vi "Control Panel.vi"() -> ()   [LabVIEW 2020]
panel:
  in  "Enable/Disable":bool
  out "Panel 8":bool
  out "Panel 7":bool
  out "Panel 6":bool
  out "Panel 5":bool
  out "Panel 4":bool
  out "Panel 3":bool
  out "Panel 2":bool
  out "Panel 1":bool
  out "Holoprojector 3":bool
  out "Holoprojector 2":bool
  out "Holoprojector 1":bool
  out "2D Picture":picture
  in  "Tab Control":enum32{"Controls", "Diagnositcs/Settings"}(tab)
  in  "Preset 1":bool
  in  "Holoprojector A":bool
  in  "Holoprojector B":bool
  in  "Holoprojector C":bool
  in  "Panel A":bool
  in  "Panel B":bool
  in  "Panel C":bool
  in  "Panel D":bool
  in  "Panel E":bool
  in  "Panel F":bool
  in  "Panel G":bool
  in  "Panel H":bool
  in  "Preset 2":bool
  in  "Preset 3":bool
  in  "Preset 4":bool
  in  "Preset 5":bool
  in  "Preset 6":bool
  in  "Preset 7":bool
  in  "Preset 8":bool
  in  "Preset 9":bool
  in  "Sound 1":bool
  in  "Sound 2":bool
  in  "Sound 3":bool
  in  "Sound 4":bool
  in  "Sound 5":bool
  out "Battery Voltage":dbl(graph)
  # "Camera Display"
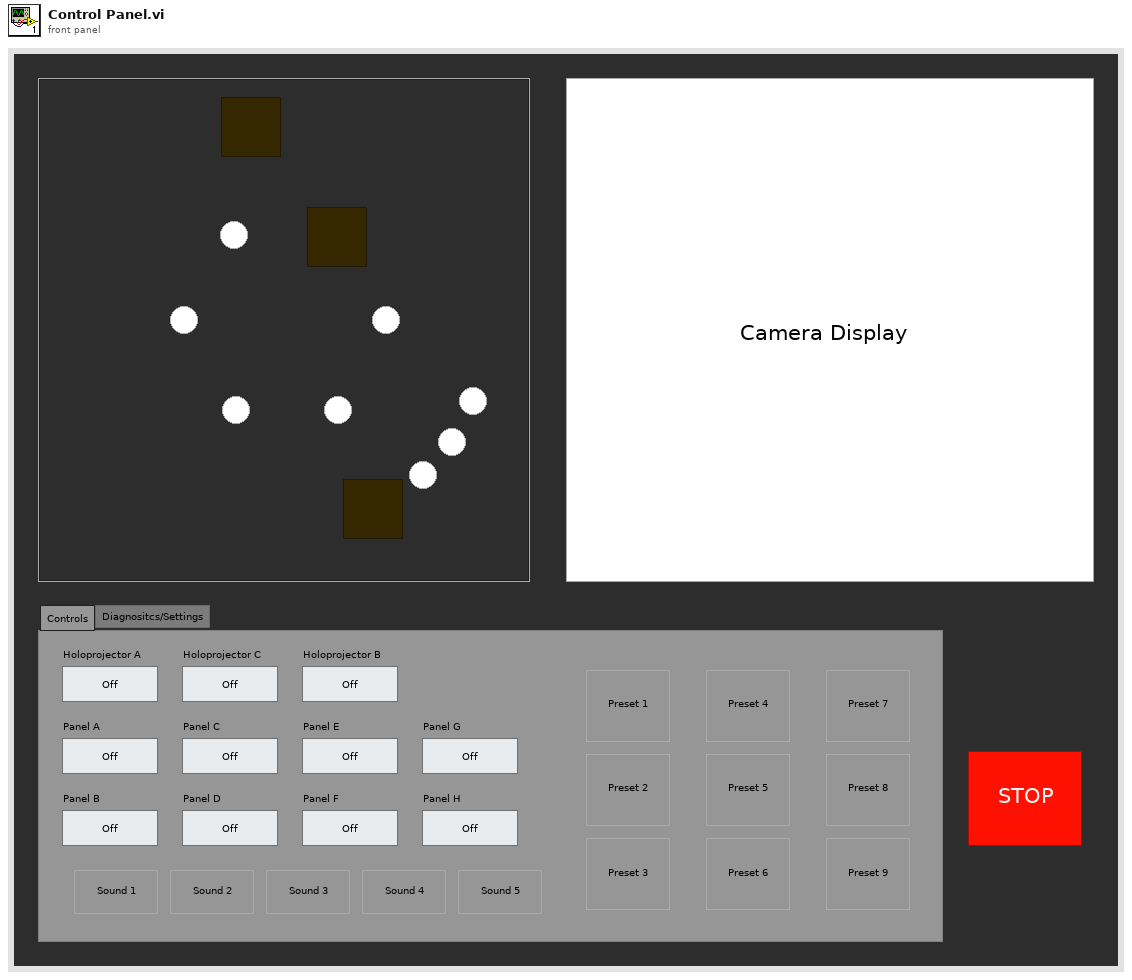
[diagram p1: front panel]
types:
  T1 = typedef "imagedata.ctl" = cluster{"image type":i32, "image depth":i32, "image":u8[], "mask":u8[], "colors":u32[], "Rectangle":cluster{"left":i16, "top":i16, "right":i16, "bottom":i16}}
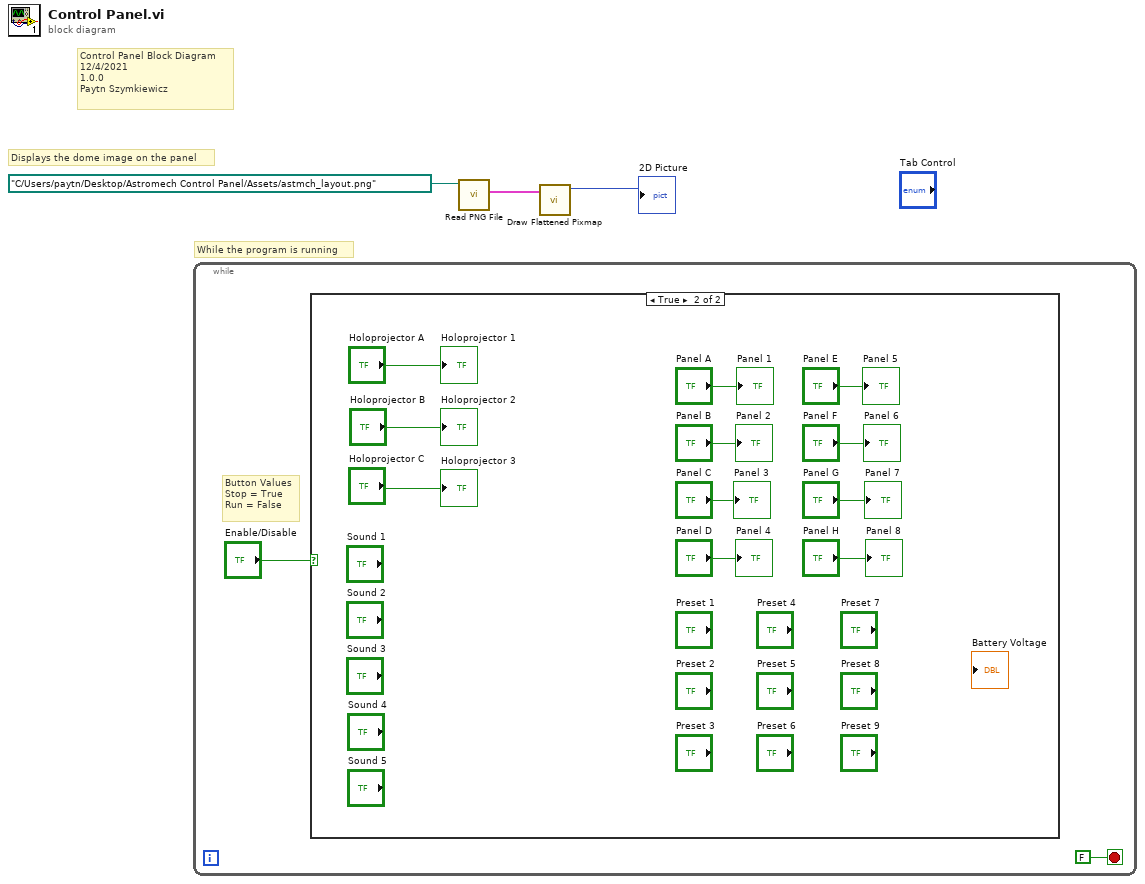
[diagram p0: block diagram]
diagram:
  # "While the program is running"
  # "Displays the dome image on the panel"
  # "Control Panel Block Diagram\n12/4/2021\n1.0.0\nPaytn Szymkiewicz"
  n1 = while {
    stop <- FALSE stop-if-true
    # "Button Values\nStop = True\nRun = False"
    n2 = case shown="True" "Enable/Disable" {
      frame False {
      }
      frame True {
        "Holoprojector 1" <- "Holoprojector A"
        "Holoprojector 2" <- "Holoprojector B"
        "Holoprojector 3" <- "Holoprojector C"
        "Panel 1" <- "Panel A"
        "Panel 2" <- "Panel B"
        "Panel 3" <- "Panel C"
        "Panel 4" <- "Panel D"
        "Panel 5" <- "Panel E"
        "Panel 6" <- "Panel F"
        "Panel 7" <- "Panel G"
        "Panel 8" <- "Panel H"
      }
    }
  }
  n3 = call <vilib>:"Read PNG File.vi"("path to PNG file"=path "C:/Users/paytn/Desktop/Astromech Control Panel/Assets/astmch_layout.png") -> ("image data"=w2:T1)  [unwired: 8 in, 2 out]
  n4 = call <vilib>:"Draw Flattened Pixmap.vi"("image data"=w2) -> ("new picture"=→"2D Picture":picture)  [unwired: 8 in]
